vi "Day 06 Part 2.vi"(11 "Input":string) -> (3 "Output":dbl format="%#.6f")   [LabVIEW 2021]
panel:
  out "Numeric":dbl
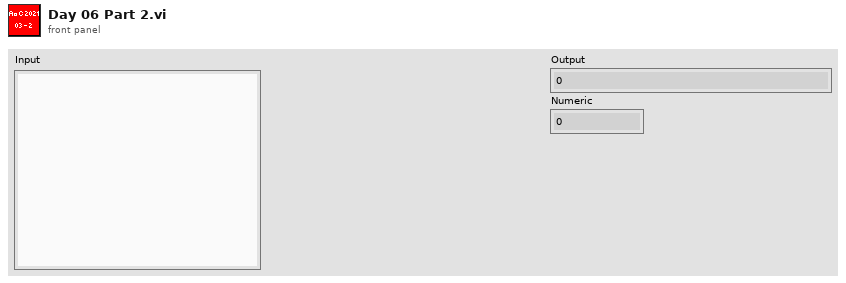
[diagram p1: front panel]
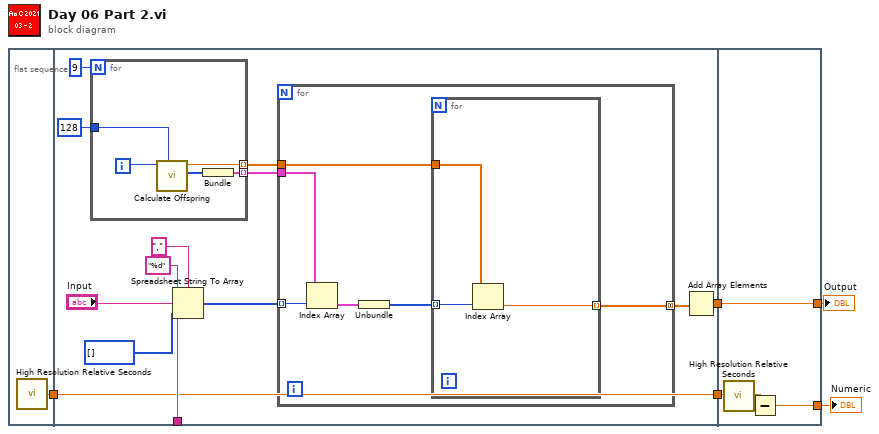
[diagram p0: block diagram]
diagram:
  n1 = flat-sequence {
    tunnel: [w7] -> w2
    tunnel: "Input" -> [w13]
    tunnel: [w9] -> w4
    tunnel: [w8] -> w3
    tunnel: w2 -> [w8]
    tunnel: [w37] -> w5
    tunnel: w4 -> [w37]
    tunnel: w3 -> [w35]
    tunnel: [w34] -> w1
    frame #0 {
      n2 = call <vilib>:"High Resolution Relative Seconds.vi"() -> ("relative seconds"=w7:dbl)
    }
    frame #1 {
      n3 = for {
        N: 9 -> [_]
        tunnel: 128 -> [w23]
        tunnel: [w22] -> w11 mode=indexing
        tunnel: [w20] -> w12 mode=indexing
        i -> [w24]
        n4 = call "Calculate Offspring.vi"("Days"=w23, "Age"=w24) -> ("Population"=w21:i8[], "Offspring"=w22:dbl)  [unwired: 8 in]
        n5 = Bundle("Population"=w21) -> (w20:cluster{"Population":i8[]})  [unwired: 1 in]
      }
      n6 = Spreadsheet String To Array(delimiter (Tab)=",", format string="%d", spreadsheet string=w13, array type (2D Dbl)=i32[] []) -> (array=w14:i32[])
      n7 = for {
        tunnel: w14 -> [w30] mode=indexing
        tunnel: w12 -> [w29]
        tunnel: w11 -> [w26]
        tunnel: [w25] -> w10 mode=concatenating
        n8 = Index Array(array=w29, index=w30) -> (element=w28:cluster{"Population":i8[]})
        n9 = Unbundle(w28) -> ("Population"=w27:i8[])
        n10 = for {
          tunnel: w27 -> [w33] mode=indexing
          tunnel: w26 -> [w32]
          tunnel: [w31] -> w25 mode=indexing
          n11 = Index Array(array=w32, index=w33) -> (element=w31:dbl)
        }
      }
      n12 = Add Array Elements(numeric array=w10) -> (sum=w9:dbl)
    }
    frame #2 {
      n13 = call <vilib>:"High Resolution Relative Seconds.vi"() -> ("relative seconds"=w36:dbl)
      n14 = Subtract(x=w36, y=w35) -> (x-y=w34:dbl)
    }
  }
  "Output" <- w5
  "Numeric" <- w1
